vi "toplevel.vi"() -> ()   [LabVIEW 2011]
uses:
  state_machine_states.ctl
  <vilib>/sound2/lvsound2.llb/Sampling Mode.ctl
  <vilib>/sound2/lvsound2.llb/Sound Data Format.ctl
  <vilib>/Analysis/4window.llb/windowTd.ctl
  <vilib>/Analysis/3filter.llb/Filter Passband Type.ctl
  global_sound_task_id.vi
  global_error_anywhere.vi
  global_parameters_changed.vi
  <vilib>/sound2/lvsound2.llb/Sound Output Set Volume (Single).vi
  global_queue.vi
  global_bool.vi
  <vilib>/measure/maspectr.llb/FFT Spectrum (Mag-Phase) for 1 Chan.vi
  <vilib>/Analysis/3filter.llb/FIR Windowed Filter (DBL).vi
  <vilib>/measure/maspectr.llb/FFT Spectrum (Mag-Phase) for 1 Chan (CDB).vi
  <vilib>/Analysis/NI_AALBase.lvlib
  <vilib>/measure/NI_MAPro.lvlib
  <vilib>/Analysis/NI_AALPro.lvlib
panel:
  out "Queue size:":i32(slide) scale=0.0..4.0 scale format="%.0p"
  out "Spectrum of the FM demodulated signal":cluster{"f0":dbl, "df":dbl, "magnitude":dbl[]}(graph)
  out "Feed snd.:":i32(slide) scale=0.0..45001.0 scale format="%.0p"
  out "Decimation:":i32(slide) scale=0.0..1.0
  out "LPF:":i32(slide) scale=0.0..1.0
  out "TCP read/write:":i32(slide) scale=0.0..1.0
  out "FM demod:":i32(slide) scale=0.0..500000.0
  in  "Frequency:":u32=100000000
  in  "Samplerate:":string(combo)="250000"
  in  "Autogain":bool=TRUE
  in  "Gain:":i32(slide)=30 min=0 max=30 scale=0.0..80.0
  in  "Device ID:":u16
  in  "Output rate:":string(combo)="50000"
  in  "Host:":string="localhost"
  in  "Play":bool
  out "RF spectrum":cluster{"f0":dbl, "df":dbl, "magnitude":dbl[]}(graph)
  in  "Port:":u16=1234
  in  "Volume:":dbl(slide)=100.0 min=0.0 max=1.0 scale=0.0..100.0
  # "I/Q input"
  # "sps"
  # "Hz"
  # "Sound output settings"
  # "Copyright (c) 2013 András Retzler"
  # "sps"
  # "(c) 2013 András Retzler"
  # "Buffer processing status"
  # "Copyright (c) 2013 András Retzler"
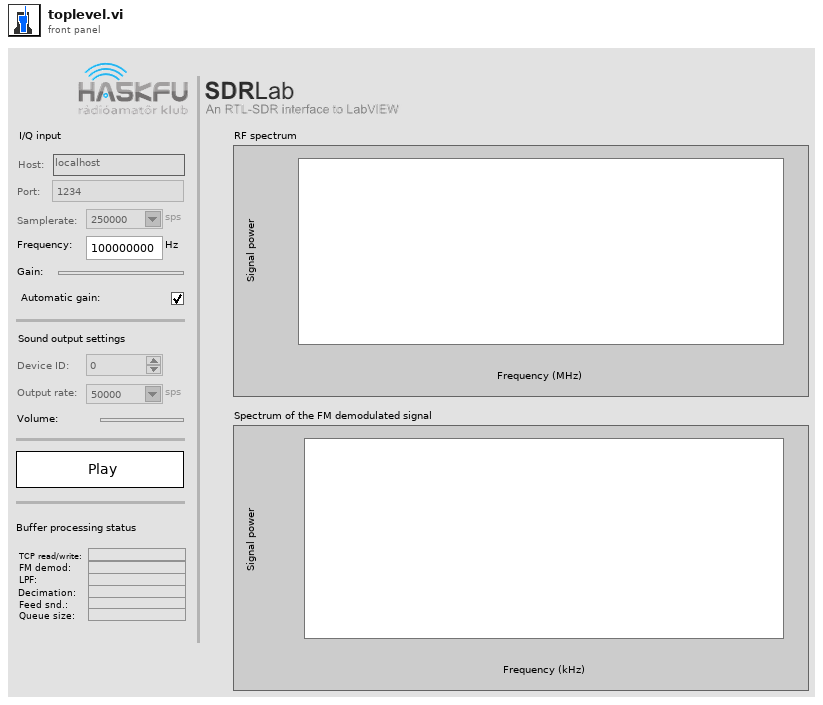
[diagram p1: front panel]
types:
  T1 = typedef "state_machine_states.ctl" = enum16{"Setup", "Play"}
  T2 = typedef "NI_AALBase.lvlib/Filter Passband Type.ctl" = enum32{"Lowpass", "Highpass", "Bandpass", "Bandstop"}
  T3 = enum8{"Enabled", "Disabled", "Disabled and Grayed Out"}
  T4 = typedef "Sampling Mode.ctl" = i32
  T5 = typedef "Sound Data Format.ctl" = cluster{"sample rate (S/s)":dbl, "number of channels":i32, "bits per sample":i32}
  T6 = typedef "Sound Output Task ID.ctl" = u32
  T7 = typedef "NI_AALPro.lvlib/windowTd.ctl" = u32
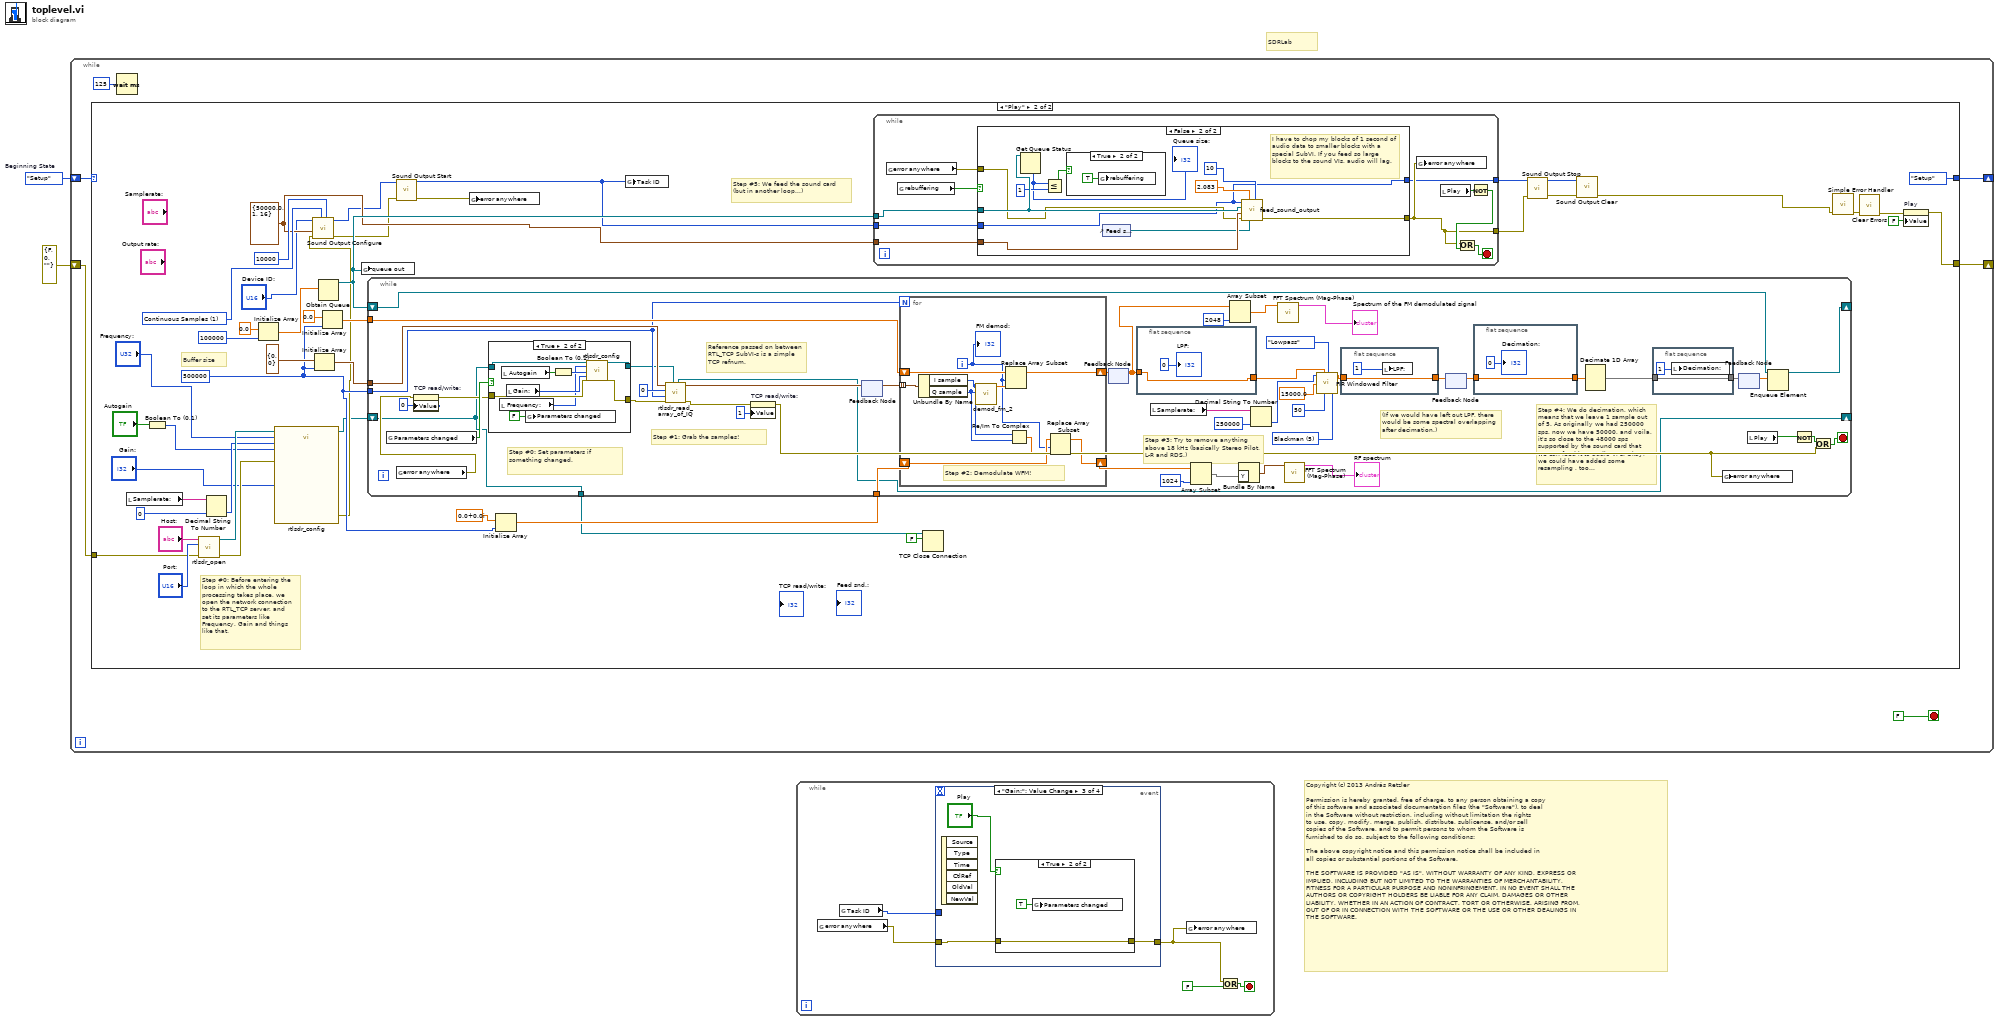
[diagram p0: block diagram]
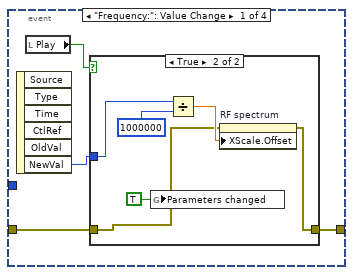
[diagram p2: hidden frame]
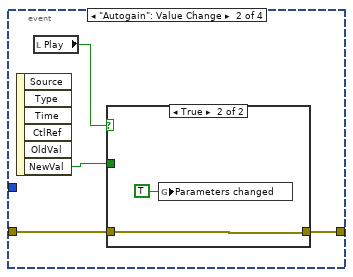
[diagram p4: hidden frame]
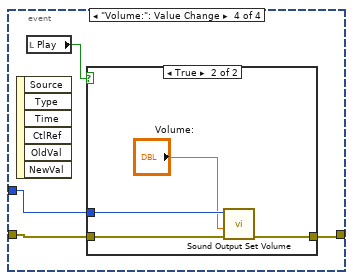
[diagram p7: hidden frame]
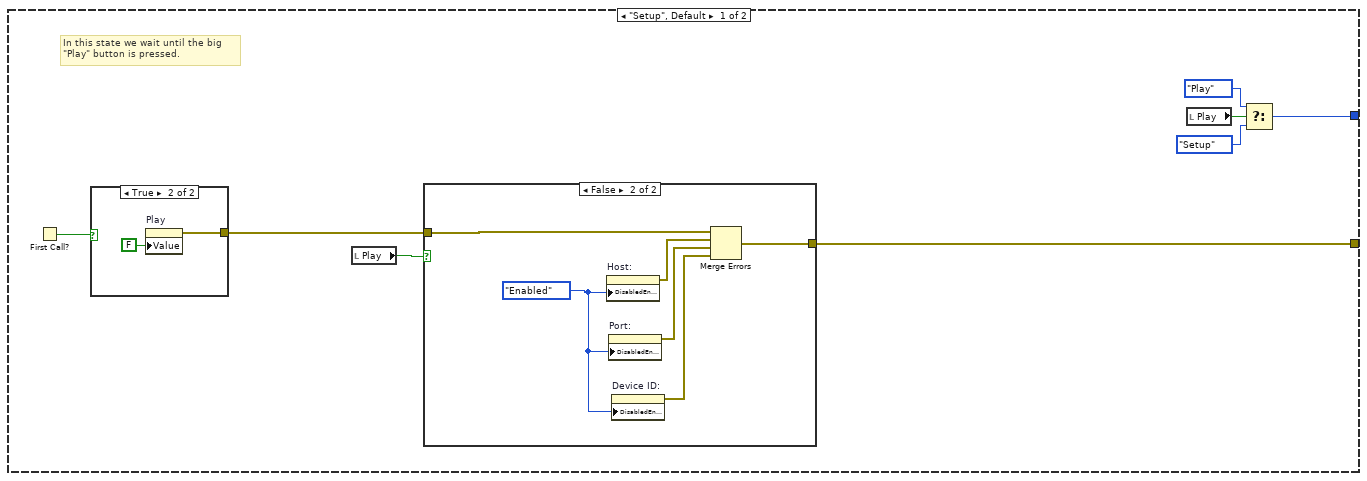
[diagram p9: hidden frame]
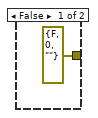
[diagram p10: hidden frame]
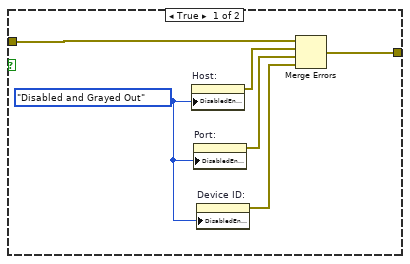
[diagram p11: hidden frame]
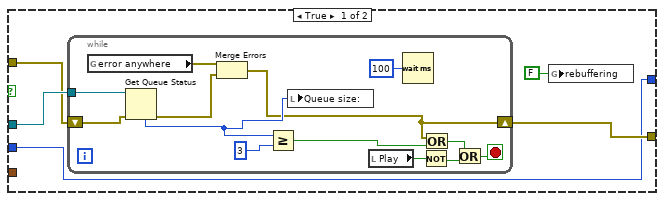
[diagram p12: hidden frame]
diagram:
  w2 = state_machine_states."Setup"  # Beginning State
  # "SDRLab"
  # "Copyright (c) 2013 András Retzler\n\nPermission is hereby granted, free of charge, to any person obtaining a copy\nof this software and associated documentation files (the \"Software\"), to deal\nin the Software without restriction, including without limitation the rights\nto use, copy, modify, merge, publish, distribute, sublicense, and/or sell\ncopies of the Software, and to permit persons to whom the Software is\nfurnished to do so, subject to the following conditions:\n\nThe above copyright notice and this permission notice shall be included in\nall copies or substantial portions of the Software.\n\nTHE SOFTWARE IS PROVIDED \"AS IS\", WITHOUT WARRANTY OF ANY KIND, EXPRESS OR\nIMPLIED, INCLUDING BUT NOT LIMITED TO THE WARRANTIES OF MERCHANTABILITY,\nFITNESS FOR A PARTICULAR PURPOSE AND NONINFRINGEMENT. IN NO EVENT SHALL THE\nAUTHORS OR COPYRIGHT HOLDERS BE LIABLE FOR ANY CLAIM, DAMAGES OR OTHER\nLIABILITY, WHETHER IN AN ACTION OF CONTRACT, TORT OR OTHERWISE, ARISING FROM,\nOUT OF OR IN CONNECTION WITH THE SOFTWARE OR THE USE OR OTHER DEALINGS IN\nTHE SOFTWARE."
  n1 = while {
    shift-right: [w8] -> _
    shift-left: w2 -> [w5]
    shift-right: [w4] -> _
    shift-left: errorcluster {"status"=FALSE, "code"=0, "source"=""} ("error constant") -> [w3]
    stop <- FALSE stop-if-true
    n2 = case shown="\"Play\"" w5 {
      tunnel: [w16 state_machine_states."Setup" ("Next State")] -> w8
      tunnel: [w9 w55] -> w4
      tunnel: w3 -> [_ w56]
      frame "Setup", Default {
        # "In this state we wait until the big \"Play\" button is pressed."
        n3 = First Call?() -> (First Call?: T/F=w11:bool)
        n4 = case shown="True" w11 {
          tunnel: [errorcluster {"status"=FALSE, "code"=0, "source"=""} ("error out") w18] -> w10
          frame False {
          }
          frame True {
            n5 = property on="Play" class="Bool (strict)"("Value"=FALSE ("Play")) -> (error out=w18:errorcluster)  [unwired: 2 in, 1 out]
          }
        }
        n6 = local read "Play"() -> (w12:bool)
        n7 = case shown="False" w12 {
          tunnel: w10 -> [w24 w30]
          tunnel: [w20 w26] -> w9
          frame True {
            w25 = T3."Disabled and Grayed Out" ("Disabled")
            n8 = property on="Host:" class="Str"("DisabledEnum"=w25) -> (error out=w23:errorcluster)  [unwired: 2 in, 1 out]
            n9 = property on="Port:" class="DigNum (strict)"("DisabledEnum"=w25) -> (error out=w22:errorcluster)  [unwired: 2 in, 1 out]
            n10 = property on="Device ID:" class="DigNum (strict)"("DisabledEnum"=w25) -> (error out=w21:errorcluster)  [unwired: 2 in, 1 out]
            n11 = Merge Errors(w24, w23, w22, w21) -> (w20:errorcluster)
          }
          frame False {
            w31 = T3."Enabled" ("Disabled")
            n12 = property on="Host:" class="Str"("DisabledEnum"=w31) -> (error out=w29:errorcluster)  [unwired: 2 in, 1 out]
            n13 = property on="Port:" class="DigNum (strict)"("DisabledEnum"=w31) -> (error out=w28:errorcluster)  [unwired: 2 in, 1 out]
            n14 = property on="Device ID:" class="DigNum (strict)"("DisabledEnum"=w31) -> (error out=w27:errorcluster)  [unwired: 2 in, 1 out]
            n15 = Merge Errors(w30, w29, w28, w27) -> (w26:errorcluster)
          }
        }
        n16 = local read "Play"() -> (w15:bool)
        n17 = Select(t=state_machine_states."Play" ("state"), s=w15, f=state_machine_states."Setup" ("state")) -> (s? t:f=w16:T1)
      }
      frame "Play" {
        w62 = u32 500000 ("Buffer")
        w67 = T4 1 items=["Finite Samples", "Continuous Samples"] ("sample mode")
        w58 = T5 {"sample rate (S/s)"=50000.0, "number of channels"=1, "bits per sample"=16} ("sound format")
        # "Step #5: We feed the sound card (but in another loop...)"
        # "Step #0: Before entering the loop in which the whole processing takes place, we open the network connection to the RTL_TCP server, and set its parameters like Frequency, Gain and things like that."
        # "Buffer size"
        n18 = local read "Samplerate:"() -> (w72:string)
        n19 = Boolean To (0,1)(Boolean="Autogain") -> (0, 1=w35:i16)
        n20 = call "rtlsdr_open.vi"("error in"=w56, "remote port"="Port:", "address"="Host:") -> ("error out"=w41:errorcluster, "ref"=w39:refnum<k5>)  [unwired: 7 in]
        n21 = Decimal String To Number(string=w72, default (0L)=0 ("default (0 I32)")) -> (number=w37:i32)  [unwired: 1 in, 1 out]
        n22 = Initialize Array(0.0 ("element"), 100000 ("dimension size")) -> (w63:dbl[])
        n23 = call "rtlsdr_config.vi"("ref in"=w39, "LO frequency"="Frequency:", "Samplerate"=w37, "Autogain"=w35, "error in"=w41, "Tuner gain by index"="Gain:") -> ("ref out"=w33:refnum<k5>, "error out"=w40:errorcluster)  [unwired: 12 in]
        n24 = call <vilib>:"Sound Output Configure.vi"("number of samples/ch"=10000, "sample mode"=w67, "error in (no error)"=w40, "sound format"=w58, "device ID"="Device ID:") -> ("error out"=w49:errorcluster, "task ID"=w47:T6)  [unwired: 5 in]
        n25 = Initialize Array(cluster{"I sample":u8, "Q sample":u8} {"I sample"=0, "Q sample"=0} ("I/Q sample cluster"), w62) -> (w69:cluster{"I sample":u8, "Q sample":u8}[])
        n26 = Obtain Queue(element data type=w63) -> (queue out=w59:refnum<queue>)  [unwired: 4 in, 2 out]
        n27 = Initialize Array(sgl 0.0 ("sample out"), w62) -> (w68:sgl[])
        n28 = global write "global_queue.vi" "queue out"(w59) -> ()
        n29 = call <vilib>:"Sound Output Start.vi"("error in (no error)"=w49, "task ID"=w47) -> ("error out"=w48:errorcluster, "task ID out"=w42:T6)  [unwired: 8 in]
        n30 = global write "global_error_anywhere.vi" "error anywhere"(w48) -> ()
        n31 = Initialize Array(cdb 0.0+0.0i ("x + iy"), w62) -> (w61:cdb[])
        n32 = while {
          tunnel: w69 -> [w159]
          tunnel: w68 -> [w158]
          tunnel: w62 -> [w157]
          shift-right: [w152] -> _
          shift-left: w59 -> [w151]
          tunnel: w61 -> [w148]
          tunnel: [w125] -> w52
          shift-right: [w124] -> _
          shift-left: w33 -> [w125]
          stop <- w134 stop-if-true
          w117 = T7 5 items=["Rectangle"=0, "Hanning"=1, "Hamming"=2, "Blackman-Harris"=3, "Exact Blackman"=4, "Blackman"=5, "Flat Top"=6, "4 Term B-Harris "=7, "7 Term B-Harris"=8, "Low Sidelobe"=9, "Blackman Nuttall"=11, "Triangle"=30, "Bartlett-Hanning"=31, "Bohman"=32, "Parzen"=33, "Welch"=34, "Kaiser"=60, "Dolph-Chebyshev"=61, "Gaussian"=62] ("window")
          # "Step #0: Set parameters if something changed."
          # "(If we would have left out LPF, there would be some spectral overlapping after decimation.)"
          # "Step #4: We do decimation, which means that we leave 1 sample out of 5. As originally we had 250000 sps, now we have 50000, and voila, it's so close to the 48000 sps supported by the sound card that we can feed it to audio VI-s. Okay, we could have added some resampling , too..."
          # "Step #3: Try to remove anything above 18 kHz (basically Stereo Pilot, L-R and RDS.)"
          # "Reference passed on between RTL_TCP SubVI-s is a simple TCP refnum."
          # "Step #1: Grab the samples!"
          n33 = global read "global_parameters_changed.vi" "Parameters changed"() -> (w128:bool)
          n34 = global read "global_error_anywhere.vi" "error anywhere"() -> (w127:errorcluster)
          n35 = property on="TCP read/write:" class="Slide (strict)"(error in=w127, "Value"=0 ("Read TCP:")) -> (error out=w126:errorcluster)  [unwired: 1 in, 1 out]
          n36 = case shown="True" w128 {
            tunnel: w125 -> [w166 w175]
            tunnel: [w166 w174] -> w132
            tunnel: w126 -> [w165 w171]
            tunnel: [w165 w172] -> w131
            frame False {
            }
            frame True {
              n37 = local read "Frequency:"() -> (w167:u32)
              n38 = local read "Autogain"() -> (w170:bool)
              n39 = local read "Gain:"() -> (w168:i32)
              n40 = global write "global_parameters_changed.vi" "Parameters changed"(FALSE ("Parameters changed")) -> ()
              n41 = Boolean To (0,1)(Boolean=w170) -> (0, 1=w169:i16)
              n42 = call "rtlsdr_config.vi"("ref in"=w175, "LO frequency"=w167, "Autogain"=w169, "Gain"=w168, "error in"=w171) -> ("ref out"=w174:refnum<k5>, "error out"=w172:errorcluster)  [unwired: 13 in]
            }
          }
          n43 = call "rtlsdr_read_array_of_IQ.vi"("ref in"=w132, "error in (no error)"=w131, "buffer size"=w157, "index"=u32 0 ("next index"), "array in"=w159) -> ("error out"=w130:errorcluster, "array out"=w145:cluster{"I sample":u8, "Q sample":u8}[], "ref out"=w124:refnum<k5>)  [unwired: 3 in, 1 out]
          n44 = property on="TCP read/write:" class="Slide (strict)"(error in=w130, "Value"=1 ("Read TCP:")) -> (error out=w129:errorcluster)  [unwired: 1 in, 1 out]
          n45 = feedback-in #1(w145) -> ()
          n46 = feedback #1() -> (w161:cluster{"I sample":u8, "Q sample":u8}[])  [unwired: 1 in]
          n47 = for {
            N: w157 -> [_]
            shift-right: [w193] -> w160
            shift-left: w158 -> [w192]
            tunnel: w161 -> [w191] mode=indexing
            shift-right: [w186] -> w140
            shift-left: w148 -> [w187]
            i -> [w184]
            # "Step #2: Demodulate WFM!"
            n48 = Unbundle By Name(w191) -> ("I sample"=w188:u8, "Q sample"=w189:u8)
            n49 = call "demod_fm_2.vi"("Q input"=w189, "I input"=w188) -> ("sample out"=w190:sgl)  [unwired: 9 in]
            n50 = Replace Array Subset(array=w192, new element=w190, index=w184) -> (w193:sgl[])
            n51 = Re/Im To Complex(1:w189, 2:w188) -> (0:w185:cdb)
            n52 = Replace Array Subset(array=w187, new element=w185, index=w184) -> (w186:cdb[])
            "FM demod:" <- w184
          }
          n53 = feedback #2() -> (w142:sgl[])  [unwired: 1 in]
          n54 = feedback-in #2(w160) -> ()
          n55 = flat-sequence {
            tunnel: [w182] -> w122
            tunnel: w142 -> [w182]
            frame #0 {
              "LPF:" <- 0 ("Get samples")
            }
          }
          n56 = local read "Samplerate:"() -> (w163:string)
          n57 = Array Subset(array=w140, length=1024) -> (w138:cdb[])  [unwired: 1 in]
          n58 = Array Subset(array=w142, length=2048) -> (w143:sgl[])  [unwired: 1 in]
          n59 = Bundle By Name("Y"=w138) -> (w137:waveform(cdb))  [unwired: 1 in]
          n60 = Decimal String To Number(string=w163, default (0L)=250000 ("default (0 I32)")) -> (number=w120:i32)  [unwired: 1 in, 1 out]
          n61 = call-poly <vilib>:"FFT Spectrum (Mag-Phase).vi"("time signal"=w143) -> ("magnitude"=→"Spectrum of the FM demodulated signal":cluster{"f0":dbl, "df":dbl, "magnitude":dbl[]})  [unwired: 6 in, 4 out]
          n62 = call-poly <vilib>:"FFT Spectrum (Mag-Phase).vi"("time signal"=w137) -> ("magnitude"=→"RF spectrum":cluster{"f0":dbl, "df":dbl, "magnitude":dbl[]})  [unwired: 6 in, 4 out]
          n63 = call-poly <vilib>:"FIR Windowed Filter.vi"("sampling freq: fs"=w120, "X"=w122, "filter type"=Filter_Passband_Type."Lowpass", "low cutoff freq: fl"=15000.0, "taps"=50 ("order"), "window"=w117) -> ("Filtered X"=w123:dbl[])  [unwired: 8 in, 1 out]
          n64 = flat-sequence {
            tunnel: w123 -> [w180]
            tunnel: [w180] -> w153
            frame #0 {
              n65 = local write "LPF:"(1 ("Get samples")) -> ()
            }
          }
          n66 = feedback #3() -> (w156:dbl[])  [unwired: 1 in]
          n67 = feedback-in #3(w153) -> ()
          n68 = flat-sequence {
            tunnel: w156 -> [w178]
            tunnel: [w178] -> w155
            frame #0 {
              "Decimation:" <- 0 ("Get samples")
            }
          }
          n69 = Decimate 1D Array(w155) -> (w133:dbl[])  [unwired: 4 out]
          n70 = flat-sequence {
            tunnel: w133 -> [w176]
            tunnel: [w176] -> w154
            frame #0 {
              n71 = local write "Decimation:"(1 ("Get samples")) -> ()
            }
          }
          n72 = global write "global_error_anywhere.vi" "error anywhere"(w129) -> ()
          n73 = feedback #4() -> (w150:dbl[])  [unwired: 1 in]
          n74 = feedback-in #4(w154) -> ()
          n75 = local read "Play"() -> (w136:bool)
          n76 = Enqueue Element(queue=w151, element=w150) -> (queue out=w152:refnum<queue>)  [unwired: 2 in, 2 out]
          n77 = Not(x=w136) -> (.not. x?=w135:bool)
          n78 = Or(x=w135, y=w129) -> (x .or. y?=w134:bool)
        }
        n79 = global write "global_sound_task_id.vi" "Task ID"(w42) -> ()
        n80 = while {
          tunnel: w59 -> [w85]
          tunnel: w42 -> [w84]
          tunnel: w58 -> [w83]
          tunnel: [w78] -> w46
          tunnel: [w77] -> w50
          stop <- w82 stop-if-true
          n81 = global read "global_error_anywhere.vi" "error anywhere"() -> (w79:errorcluster)
          n82 = global read "global_bool.vi" "rebuffering"() -> (w86:bool)
          n83 = case shown="False" w86 {
            tunnel: [w89 w115] -> w78
            tunnel: w85 -> [w90 w114]
            tunnel: w84 -> [w87 w105]
            tunnel: w83 -> [_ w113]
            tunnel: w79 -> [w88 w106]
            tunnel: [w87 w105] -> w77
            frame True {
              n84 = while {
                tunnel: w90 -> [w100]
                shift-right: [w97] -> w89
                shift-left: w88 -> [w101]
                stop <- w93 stop-if-true
                n85 = global read "global_error_anywhere.vi" "error anywhere"() -> (w99:errorcluster)
                n86 = Get Queue Status(queue=w100, error in (no error)=w101) -> (error out=w98:errorcluster, # elements in queue=w103:i32)  [unwired: 1 in, 6 out]
                n87 = Merge Errors(w99, w98) -> (w97:errorcluster)
                n88 = Greater Or Equal?(x=w103, y=3) -> (x >= y?=w102:bool)
                n89 = local write "Queue size:"(w103) -> ()
                n90 = local read "Play"() -> (w95:bool)
                n91 = Wait (ms)(milliseconds to wait=u32 100) -> ()  [unwired: 1 out]
                n92 = Not(x=w95) -> (.not. x?=w92:bool)
                n93 = Or(x=w97, y=w102) -> (x .or. y?=w94:bool)
                n94 = Or(x=w94, y=w92) -> (x .or. y?=w93:bool)
              }
              n95 = global write "global_bool.vi" "rebuffering"(FALSE ("rebuffering")) -> ()
            }
            frame False {
              # "I have to chop my blocks of 1 second of audio data to smaller blocks with a special SubVI. If you feed so large blocks to the sound VIs, audio will lag."
              n96 = Get Queue Status(queue=w114) -> (# elements in queue=w108:i32)  [unwired: 2 in, 7 out]
              "Queue size:" <- w108
              n97 = Less Or Equal?(x=w108, y=1) -> (x <= y?=w107:bool)
              n98 = case shown="True" w107 {
                frame False {
                }
                frame True {
                  n99 = global write "global_bool.vi" "rebuffering"(TRUE ("rebuffering")) -> ()
                }
              }
              n100 = control-ref of="Feed snd.:"() -> (w110:refnum<vi>)
              n101 = call "feed_sound_output.vi"("Output buffer feeds [1/sec]"=u16 10, "Ctl Refnum"=w110, "Input buffer length [sec]"=2.083, "error in (no error)"=w106, "sound format"=w113, "Queue"=w114, "task ID"=w105) -> ("error out"=w115:errorcluster)  [unwired: 4 in]
            }
          }
          n102 = global write "global_error_anywhere.vi" "error anywhere"(w78) -> ()
          n103 = local read "Play"() -> (w81:bool)
          n104 = Not(x=w81) -> (.not. x?=w80:bool)
          n105 = Or(x=w78, y=w80) -> (x .or. y?=w82:bool)
        }
        n106 = TCP Close Connection(connection ID=w52, abort (F)=FALSE) -> ()  [unwired: 1 in, 2 out]
        n107 = call <vilib>:"Sound Output Stop.vi"("error in (no error)"=w46, "task ID"=w50) -> ("error out"=w44:errorcluster, "task ID out"=w45:T6)  [unwired: 8 in]
        n108 = call <vilib>:"Sound Output Clear.vi"("error in (no error)"=w44, "task ID"=w45) -> ("error out"=w43:errorcluster)  [unwired: 9 in]
        n109 = call <vilib>:"Simple Error Handler.vi"("error in (no error)"=w43) -> ("error out"=w54:errorcluster)  [unwired: 4 in, 4 out]
        n110 = call <vilib>:"Clear Errors.vi"("error in (no error)"=w54) -> ("error out"=w53:errorcluster)  [unwired: 6 in]
        n111 = property on="Play" class="Bool (strict)"(error in=w53, "Value"=FALSE ("Play")) -> (error out=w55:errorcluster)  [unwired: 1 in, 1 out]
      }
    }
    n112 = Wait (ms)(milliseconds to wait=u32 125) -> ()  [unwired: 1 out]
  }
  n113 = while {
    stop <- w197 stop-if-true
    n114 = global read "global_error_anywhere.vi" "error anywhere"() -> (w195:errorcluster)
    n115 = global read "global_sound_task_id.vi" "Task ID"() -> (w194:T6)
    n116 = event shown="[2] \"Gain:\": Value Change" {
      selector: _ -> [_ _ _ _]
      dyn-events: _ -> [_ _ _ _]
      timeout: _ -> [_ _ _ _]
      tunnel: w195 -> [w200 w213 w219 w225]
      tunnel: [w202 w212 w218 w226] -> w196
      tunnel: w194 -> [_ _ _ w224]
      event "Frequency:": Value Change {
        n117 = event-data() -> ("NewVal"=w201:u32)  [unwired: 1 in, 5 out]
        n118 = local read "Play"() -> (w199:bool)
        n119 = case shown="True" w199 {
          tunnel: [w203 w206] -> w202
          tunnel: w201 -> [_ w207]
          tunnel: w200 -> [w203 w205]
          frame False {
          }
          frame True {
            n120 = global write "global_parameters_changed.vi" "Parameters changed"(TRUE ("Parameters changed")) -> ()
            n121 = Divide(x=w207, y=u32 1000000) -> (x/y=w208:dbl)
            n122 = property on="RF spectrum" class="WFGraph (strict)"(error in=w205, "XScale.Offset"=w208) -> (error out=w206:errorcluster)  [unwired: 1 in, 1 out]
          }
        }
      }
      event "Autogain": Value Change {
        n123 = event-data() -> ("NewVal"=w211:bool)  [unwired: 1 in, 5 out]
        n124 = local read "Play"() -> (w210:bool)
        n125 = case shown="True" w210 {
          tunnel: w213 -> [w214 w216]
          tunnel: [w214 w216] -> w212
          tunnel: w211 -> [_ _]
          frame False {
          }
          frame True {
            n126 = global write "global_parameters_changed.vi" "Parameters changed"(TRUE ("Parameters changed")) -> ()
          }
        }
      }
      event "Gain:": Value Change {
        n127 = event-data() -> ()  [unwired: 1 in, 6 out]
        n128 = case shown="True" "Play" {
          tunnel: w219 -> [w220 w222]
          tunnel: [w220 w222] -> w218
          frame False {
          }
          frame True {
            n129 = global write "global_parameters_changed.vi" "Parameters changed"(TRUE ("Parameters changed")) -> ()
          }
        }
      }
      event "Volume:": Value Change {
        n130 = event-data() -> ()  [unwired: 1 in, 6 out]
        n131 = local read "Play"() -> (w223:bool)
        n132 = case shown="True" w223 {
          tunnel: [w227 w231] -> w226
          tunnel: w225 -> [w227 w230]
          tunnel: w224 -> [_ w229]
          frame False {
          }
          frame True {
            n133 = call-poly <vilib>:"Sound Output Set Volume.vi"("error in (no error)"=w230, "volume"="Volume:", "task ID"=w229) -> ("error out"=w231:errorcluster)  [unwired: 7 in, 1 out]
          }
        }
      }
    }
    n134 = global write "global_error_anywhere.vi" "error anywhere"(w196) -> ()
    n135 = Or(x=w196, y=FALSE) -> (x .or. y?=w197:bool)
  }
